vi "RTS Date and Time Adjustment.vi"(11 "Chamber 1 Socket":string[](array[string])) -> (3 "Array":dbl[][](array[numeric]))   [LabVIEW 2016]
panel:
  # "Combine index 0 and 1..into a time stamp and place in index 1."
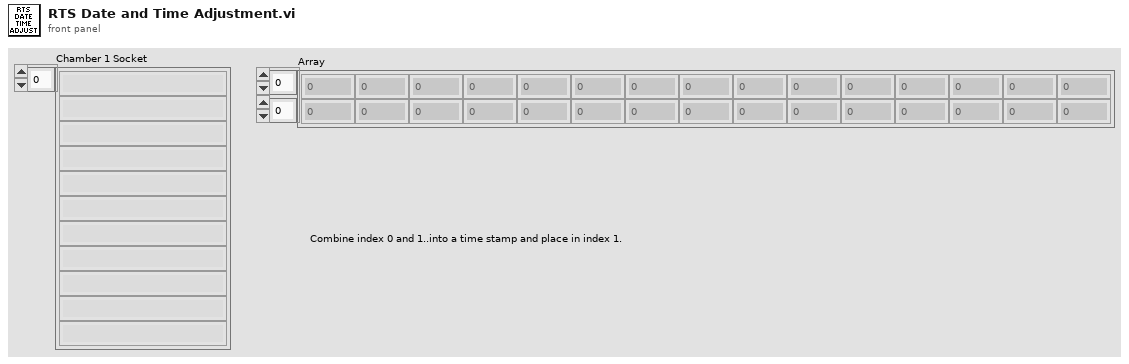
[diagram p1: front panel]
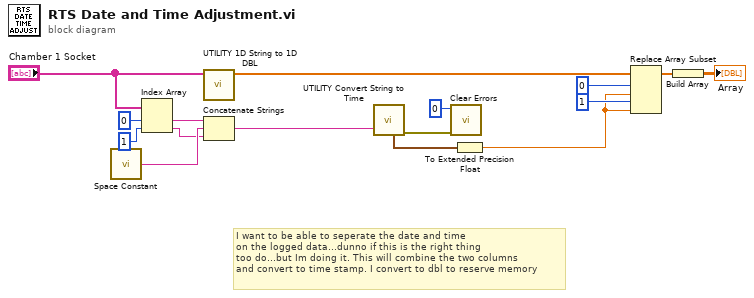
[diagram p0: block diagram]
diagram:
  # "I want to be able to seperate the date and time\non the logged data...dunno if this is the right thing\ntoo do...but Im doing it. This will combine the two columns\nand convert to time stamp. I convert to dbl to reserve memory"
  n1 = call <vilib>:"Space Constant.vi"() -> ("String"=w11:string)
  n2 = Index Array(array="Chamber 1 Socket", index #1=0 ("index"), index #2=1 ("index")) -> (element #1=w12:string, element #2=w10:string)
  n3 = call "UTILITY 1D String to 1D DBL.vi"("Save Data"="Chamber 1 Socket") -> ("DBL"=w9:dbl[])  [unwired: 10 in]
  n4 = Concatenate Strings(w12, w11, w10) -> (w6:string)
  n5 = call "UTILITY Convert String to Time.vi"("date/time string"=w6) -> ("Error Out"=w4:errorcluster, "Resulting Time Stamp"=w5:timestamp)  [unwired: 8 in, 1 out]
  n6 = call <vilib>:"Clear Errors.vi"("error in (no error)"=w4, "specific error code to clear (0: all)"=0) -> ()  [unwired: 4 in, 2 out]
  n7 = To Extended Precision Float(1:w5) -> (0:w1:ext)
  n8 = Replace Array Subset(array=w9, new element #1=w1, index #1=0 ("index"), new element #2=w1, index #2=1 ("index")) -> (w7:dbl[])
  n9 = Build Array(w7) -> (→"Array":dbl[][])
